vi "串口自动测试.vi"(9 "RS485选择":bool, 11 "RS232选择":bool) -> ()   [LabVIEW 2010]
uses:
  <vilib>/Instr/_visa.llb/VISA Configure Serial Port (Instr).vi
  全局量/试验配置信息.vi
  全局量/自动测试结果.vi
panel:
  in  "第2路RS485":string
  in  "第1路RS485":string
  in  "第2路RS232":string
  in  "第1路RS232":string
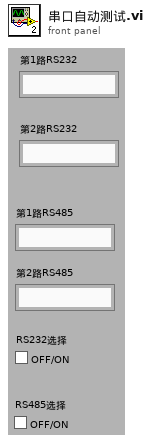
[diagram p1: front panel]
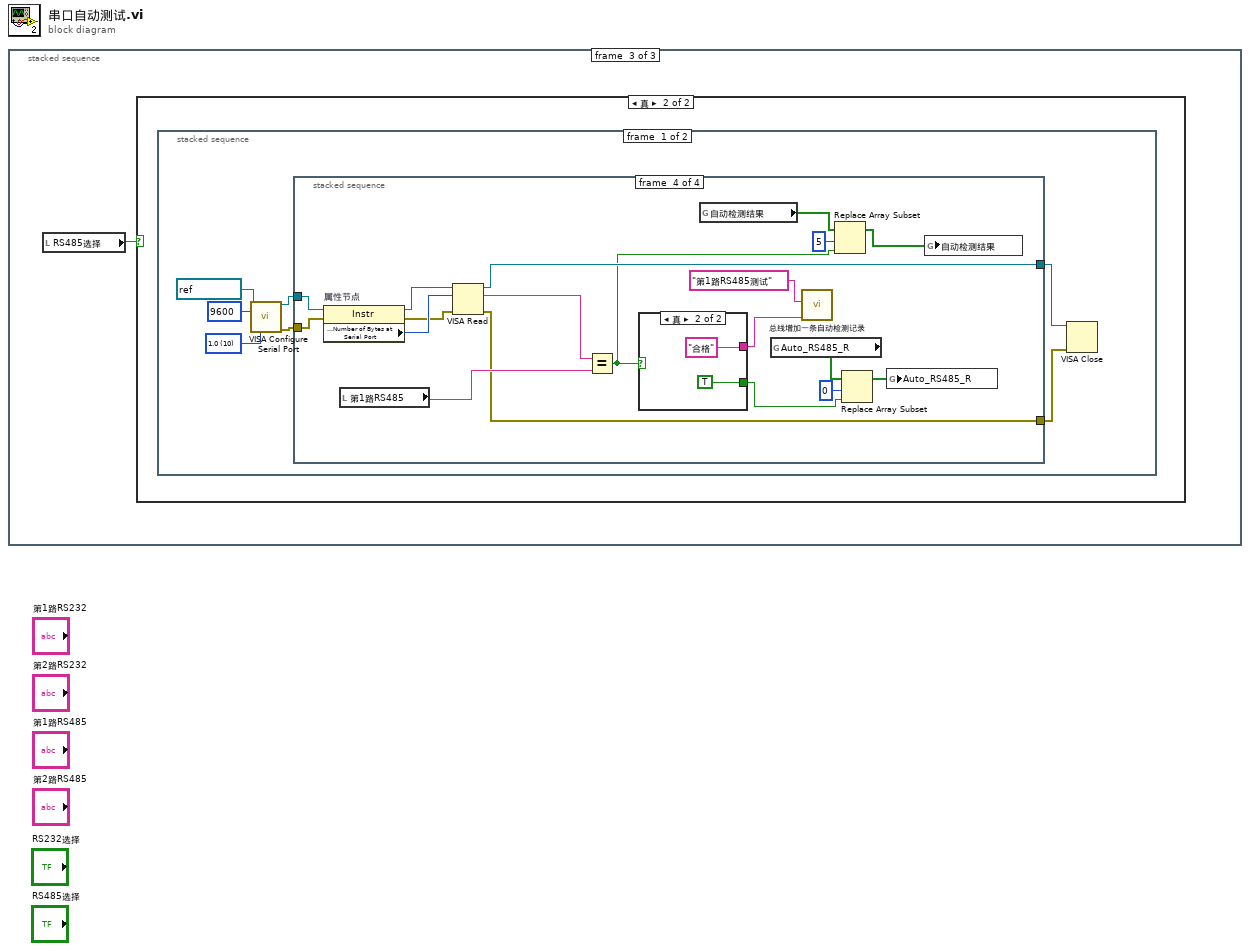
[diagram p0: block diagram]
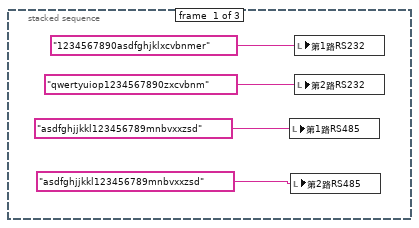
[diagram p2: hidden frame]
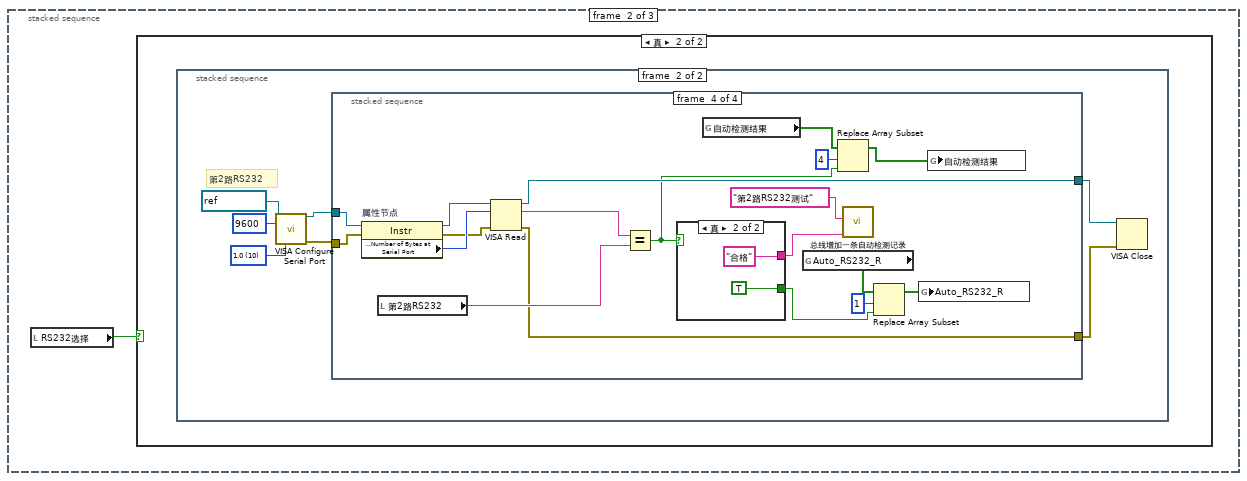
[diagram p3: hidden frame]
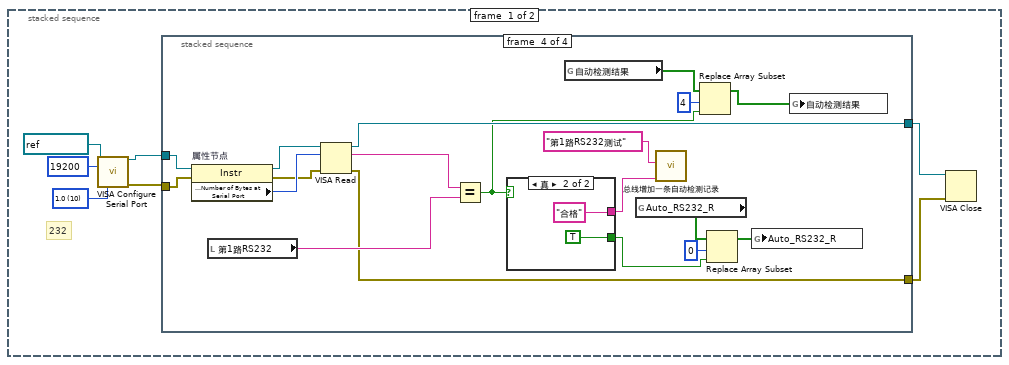
[diagram p5: hidden frame]
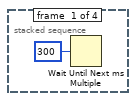
[diagram p6: hidden frame]
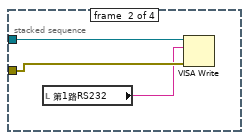
[diagram p7: hidden frame]
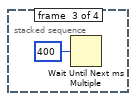
[diagram p8: hidden frame]
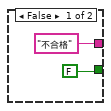
[diagram p9: hidden frame]
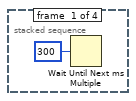
[diagram p10: hidden frame]
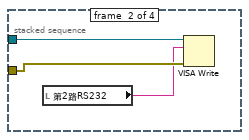
[diagram p11: hidden frame]
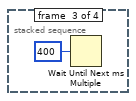
[diagram p12: hidden frame]
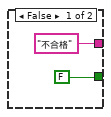
[diagram p13: hidden frame]
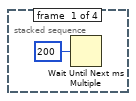
[diagram p15: hidden frame]
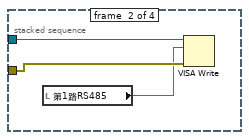
[diagram p16: hidden frame]
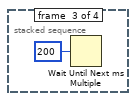
[diagram p17: hidden frame]
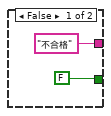
[diagram p18: hidden frame]
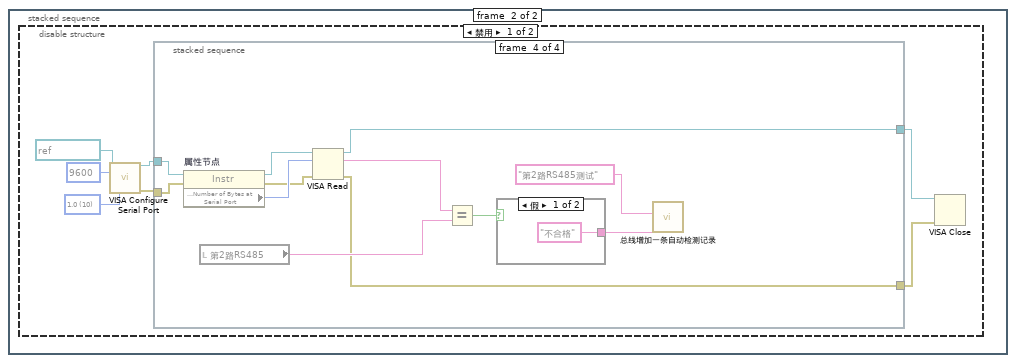
[diagram p19: hidden frame]
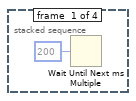
[diagram p20: hidden frame]
diagram:
  n1 = stacked-sequence {
    frame #0 {
      n2 = local write "第1路RS485"("asdfghjjkkl123456789mnbvxxzsd" ("发送字符串_3")) -> ()
      n3 = local write "第2路RS485"("asdfghjjkkl123456789mnbvxxzsd" ("发送字符串_3")) -> ()
      n4 = local write "第1路RS232"("1234567890asdfghjklxcvbnmer" ("发送字符串_1")) -> ()
      n5 = local write "第2路RS232"("qwertyuiop1234567890zxcvbnm" ("发送字符串_2")) -> ()
    }
    frame #1 {
      n6 = local read "RS232选择"() -> (w5:bool)
      n7 = case shown="真" w5 {
        frame False {
        }
        frame True {
          n8 = stacked-sequence {
            frame #0 {
              w8 = u16 10 items=["1.0"=10, "1.5"=15, "2.0"=20] ("stop bits (10: 1 bit)")
              # "232"
              n9 = call-poly "VISA Configure Serial Port"("VISA resource name"=refnum<visa-resource-name> "COM1", "baud rate (9600)"=u32 19200, "stop bits (10: 1 bit)"=w8) -> ("VISA resource name out"=w7:refnum<visa-resource-name>, "error out"=w6:errorcluster)  [unwired: 11 in]
              n10 = stacked-sequence {
                tunnel: w7 -> [_ w16 _ w30]
                tunnel: w6 -> [_ w15 _ w29]
                tunnel: [_ _ _ w32] -> w12
                tunnel: [_ _ _ w31] -> w11
                frame #0 {
                  n11 = Wait Until Next ms Multiple(millisecond multiple=u32 300 ("毫秒倍数")) -> ()  [unwired: 1 out]
                }
                frame #1 {
                  n12 = local read "第1路RS232"() -> (w14:string)
                  n13 = VISA Write(VISA resource name=w16, write buffer=w14, error in (no error)=w15) -> ()  [unwired: 3 out]
                }
                frame #2 {
                  n14 = Wait Until Next ms Multiple(millisecond multiple=u32 400 ("毫秒倍数")) -> ()  [unwired: 1 out]
                }
                frame #3 {
                  n15 = property on="属性节点" class="Instr"(reference=w30, error in=w29) -> (reference out=w36:refnum<visa-resource-name>, error out=w34:errorcluster, "Serial Settings:Number of Bytes at Serial Port"=w35:u32)
                  n16 = local read "第1路RS232"() -> (w33:string)
                  n17 = VISA Read(VISA resource name=w36, byte count=w35, error in (no error)=w34) -> (VISA resource name out=w32:refnum<visa-resource-name>, read buffer=w28:string, error out=w31:errorcluster)  [unwired: 1 out]
                  n18 = Equal?(x=w28, y=w33) -> (x = y?=w18:bool)
                  n19 = case shown="真" w18 {
                    tunnel: ["不合格" "合格"] -> w26
                    tunnel: [FALSE TRUE] -> w22
                    frame False {
                    }
                    frame True {
                    }
                  }
                  n20 = global read "试验配置信息.vi" "自动检测结果"() -> (w19:bool[])
                  n21 = global read "自动测试结果.vi" "Auto_RS232_R"() -> (w25:bool[])
                  n22 = call "总线增加一条自动检测记录.vi"("测试结果"=w26, "测试内容"="第1路RS232测试") -> ()  [unwired: 10 in]
                  n23 = Replace Array Subset(array=w19, new element=w18, index=4 ("索引")) -> (w20:bool[])
                  n24 = Replace Array Subset(array=w25, new element=w22, index=0 ("索引")) -> (w24:bool[])
                  n25 = global write "自动测试结果.vi" "Auto_RS232_R"(w24) -> ()
                  n26 = global write "试验配置信息.vi" "自动检测结果"(w20) -> ()
                }
              }
              n27 = VISA Close(VISA resource name=w12, error in (no error)=w11) -> ()  [unwired: 1 out]
            }
            frame #1 {
              w43 = u16 10 items=["1.0"=10, "1.5"=15, "2.0"=20] ("stop bits (10: 1 bit)")
              # "第2路RS232"
              n28 = call-poly "VISA Configure Serial Port"("VISA resource name"=refnum<visa-resource-name> "COM3", "baud rate (9600)"=u32 9600, "stop bits (10: 1 bit)"=w43) -> ("VISA resource name out"=w46:refnum<visa-resource-name>, "error out"=w47:errorcluster)  [unwired: 11 in]
              n29 = stacked-sequence {
                tunnel: w46 -> [_ w51 _ w65]
                tunnel: w47 -> [_ w50 _ w64]
                tunnel: [_ _ _ w67] -> w41
                tunnel: [_ _ _ w66] -> w42
                frame #0 {
                  n30 = Wait Until Next ms Multiple(millisecond multiple=u32 300 ("毫秒倍数")) -> ()  [unwired: 1 out]
                }
                frame #1 {
                  n31 = local read "第2路RS232"() -> (w49:string)
                  n32 = VISA Write(VISA resource name=w51, write buffer=w49, error in (no error)=w50) -> ()  [unwired: 3 out]
                }
                frame #2 {
                  n33 = Wait Until Next ms Multiple(millisecond multiple=u32 400 ("毫秒倍数")) -> ()  [unwired: 1 out]
                }
                frame #3 {
                  n34 = property on="属性节点" class="Instr"(reference=w65, error in=w64) -> (reference out=w71:refnum<visa-resource-name>, error out=w69:errorcluster, "Serial Settings:Number of Bytes at Serial Port"=w70:u32)
                  n35 = local read "第2路RS232"() -> (w68:string)
                  n36 = VISA Read(VISA resource name=w71, byte count=w70, error in (no error)=w69) -> (VISA resource name out=w67:refnum<visa-resource-name>, read buffer=w61:string, error out=w66:errorcluster)  [unwired: 1 out]
                  n37 = Equal?(x=w61, y=w68) -> (x = y?=w53:bool)
                  n38 = case shown="真" w53 {
                    tunnel: ["不合格" "合格"] -> w62
                    tunnel: [FALSE TRUE] -> w57
                    frame False {
                    }
                    frame True {
                    }
                  }
                  n39 = global read "试验配置信息.vi" "自动检测结果"() -> (w54:bool[])
                  n40 = global read "自动测试结果.vi" "Auto_RS232_R"() -> (w60:bool[])
                  n41 = Replace Array Subset(array=w54, new element=w53, index=4 ("索引")) -> (w55:bool[])
                  n42 = call "总线增加一条自动检测记录.vi"("测试结果"=w62, "测试内容"="第2路RS232测试") -> ()  [unwired: 10 in]
                  n43 = Replace Array Subset(array=w60, new element=w57, index=1 ("索引")) -> (w59:bool[])
                  n44 = global write "自动测试结果.vi" "Auto_RS232_R"(w59) -> ()
                  n45 = global write "试验配置信息.vi" "自动检测结果"(w55) -> ()
                }
              }
              n46 = VISA Close(VISA resource name=w41, error in (no error)=w42) -> ()  [unwired: 1 out]
            }
          }
        }
      }
    }
    frame #2 {
      n47 = local read "RS485选择"() -> (w76:bool)
      n48 = case shown="真" w76 {
        frame False {
        }
        frame True {
          n49 = stacked-sequence {
            frame #0 {
              w81 = u16 10 items=["1.0"=10, "1.5"=15, "2.0"=20] ("stop bits (10: 1 bit)")
              n50 = call-poly "VISA Configure Serial Port"("VISA resource name"=refnum<visa-resource-name> "COM4", "baud rate (9600)"=u32 9600, "stop bits (10: 1 bit)"=w81) -> ("VISA resource name out"=w78:refnum<visa-resource-name>, "error out"=w77:errorcluster)  [unwired: 11 in]
              n51 = stacked-sequence {
                tunnel: w78 -> [_ w87 _ w101]
                tunnel: w77 -> [_ w86 _ w100]
                tunnel: [_ _ _ w103] -> w83
                tunnel: [_ _ _ w102] -> w82
                frame #0 {
                  n52 = Wait Until Next ms Multiple(millisecond multiple=u32 200 ("毫秒倍数")) -> ()  [unwired: 1 out]
                }
                frame #1 {
                  n53 = local read "第1路RS485"() -> (w85:string)
                  n54 = VISA Write(VISA resource name=w87, write buffer=w85, error in (no error)=w86) -> ()  [unwired: 3 out]
                }
                frame #2 {
                  n55 = Wait Until Next ms Multiple(millisecond multiple=u32 200 ("毫秒倍数")) -> ()  [unwired: 1 out]
                }
                frame #3 {
                  n56 = property on="属性节点" class="Instr"(reference=w101, error in=w100) -> (reference out=w107:refnum<visa-resource-name>, error out=w105:errorcluster, "Serial Settings:Number of Bytes at Serial Port"=w106:u32)
                  n57 = local read "第1路RS485"() -> (w104:string)
                  n58 = VISA Read(VISA resource name=w107, byte count=w106, error in (no error)=w105) -> (VISA resource name out=w103:refnum<visa-resource-name>, read buffer=w99:string, error out=w102:errorcluster)  [unwired: 1 out]
                  n59 = Equal?(x=w99, y=w104) -> (x = y?=w89:bool)
                  n60 = case shown="真" w89 {
                    tunnel: ["不合格" "合格"] -> w97
                    tunnel: [FALSE TRUE] -> w93
                    frame False {
                    }
                    frame True {
                    }
                  }
                  n61 = global read "试验配置信息.vi" "自动检测结果"() -> (w90:bool[])
                  n62 = global read "自动测试结果.vi" "Auto_RS485_R"() -> (w96:bool[])
                  n63 = call "总线增加一条自动检测记录.vi"("测试结果"=w97, "测试内容"="第1路RS485测试") -> ()  [unwired: 10 in]
                  n64 = Replace Array Subset(array=w90, new element=w89, index=5 ("索引")) -> (w91:bool[])
                  n65 = Replace Array Subset(array=w96, new element=w93, index=0 ("索引")) -> (w95:bool[])
                  n66 = global write "自动测试结果.vi" "Auto_RS485_R"(w95) -> ()
                  n67 = global write "试验配置信息.vi" "自动检测结果"(w91) -> ()
                }
              }
              n68 = VISA Close(VISA resource name=w83, error in (no error)=w82) -> ()  [unwired: 1 out]
            }
            frame #1 {
              n69 = disable-structure shown="禁用" {
                frame Disabled {
                  w118 = u16 10 items=["1.0"=10, "1.5"=15, "2.0"=20] ("stop bits (10: 1 bit)")
                  n70 = call-poly "VISA Configure Serial Port"("VISA resource name"=refnum<visa-resource-name> "COM5", "baud rate (9600)"=u32 9600, "stop bits (10: 1 bit)"=w118) -> ("VISA resource name out"=w113:refnum<visa-resource-name>, "error out"=w112:errorcluster)  [unwired: 11 in]
                  n71 = stacked-sequence {
                    tunnel: w113 -> [_ w122 _ w128]
                    tunnel: w112 -> [_ w121 _ w127]
                    tunnel: [_ _ _ w130] -> w115
                    tunnel: [_ _ _ w129] -> w114
                    frame #0 {
                      n72 = Wait Until Next ms Multiple(millisecond multiple=u32 200 ("毫秒倍数")) -> ()  [unwired: 1 out]
                    }
                    frame #1 {
                      n73 = local read "第2路RS485"() -> (w120:string)
                      n74 = VISA Write(VISA resource name=w122, write buffer=w120, error in (no error)=w121) -> ()  [unwired: 3 out]
                    }
                    frame #2 {
                      n75 = Wait Until Next ms Multiple(millisecond multiple=u32 200 ("毫秒倍数")) -> ()  [unwired: 1 out]
                    }
                    frame #3 {
                      n76 = property on="属性节点" class="Instr"(reference=w128, error in=w127) -> (reference out=w134:refnum<visa-resource-name>, error out=w132:errorcluster, "Serial Settings:Number of Bytes at Serial Port"=w133:u32)
                      n77 = local read "第2路RS485"() -> (w131:string)
                      n78 = VISA Read(VISA resource name=w134, byte count=w133, error in (no error)=w132) -> (VISA resource name out=w130:refnum<visa-resource-name>, read buffer=w126:string, error out=w129:errorcluster)  [unwired: 1 out]
                      n79 = Equal?(x=w126, y=w131) -> (x = y?=w135:bool)
                      n80 = case shown="假" w135 {
                        tunnel: ["不合格" "合格"] -> w124
                        frame False {
                        }
                        frame True {
                        }
                      }
                      n81 = call "总线增加一条自动检测记录.vi"("测试结果"=w124, "测试内容"="第2路RS485测试") -> ()  [unwired: 10 in]
                    }
                  }
                  n82 = VISA Close(VISA resource name=w115, error in (no error)=w114) -> ()  [unwired: 1 out]
                }
                frame Enabled {
                }
              }
            }
          }
        }
      }
    }
  }
